vi "CalibrationData.vi"(1 "CalData In":dbl[][](array[numeric])) -> (0 "CalData Out":dbl[][](array[numeric]))   [LabVIEW 2015]
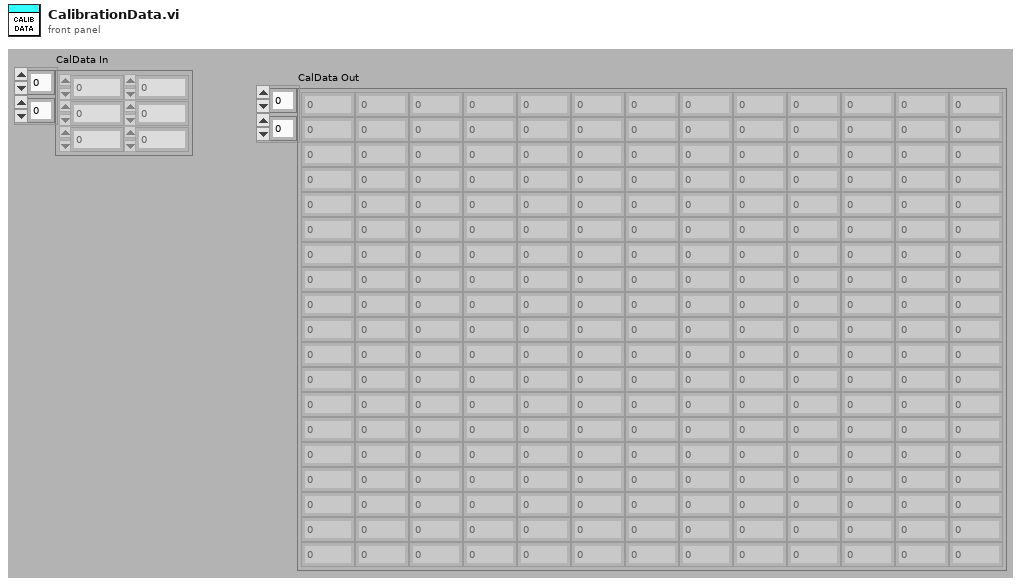
[diagram p1: front panel]
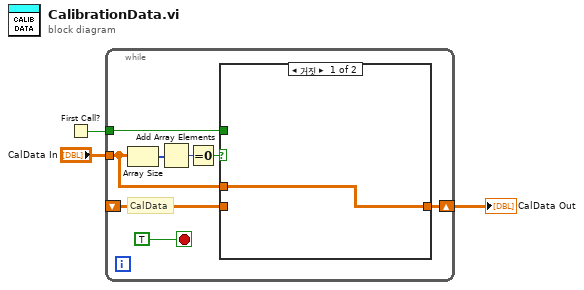
[diagram p0: block diagram]
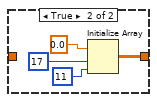
[diagram p3: hidden frame]
diagram:
  n1 = First Call?() -> (First Call?: T/F=w2:bool)
  n2 = while {
    shift-right: [w11] -> w1
    shift-left: _ -> [w10]
    tunnel: "CalData In" -> [w8]
    tunnel: w2 -> [w4]
    stop <- TRUE stop-if-true
    # "CalData"
    n3 = Array Size(array=w8) -> (size(s)=w7:i32[])
    n4 = Add Array Elements(numeric array=w7) -> (sum=w6:i32)
    n5 = Equal To 0?(x=w6) -> (x = 0?=w5:bool)
    n6 = case shown="거짓" w5 {
      tunnel: [w12 w15] -> w11
      tunnel: w10 -> [_ w14]
      tunnel: w8 -> [w12 _]
      tunnel: w4 -> [_ w13]
      frame False {
      }
      frame True {
        n7 = case shown="거짓" w13 {
          tunnel: [w16 w18] -> w15
          tunnel: w14 -> [w16 _]
          frame False {
          }
          frame True {
            n8 = Initialize Array(0.0 ("Numeric"), 17 ("dimension size"), 11 ("dimension size")) -> (w18:dbl[][])
          }
        }
      }
    }
  }
  "CalData Out" <- w1
